vi "INIT SetPortProperties.vi"(8 "error in (no error)":errorcluster, 11 "Device Item Ref in":T1 format="%.0x") -> (0 "error out":errorcluster, 3 "Device Item Ref out":T1 format="%.0x")   [LabVIEW 2018, in "CAN Gateway System Explorer.lvlib"]
uses:
  CAN Gateway System Explorer.lvlib
  <vilib>/NI Veristand/Custom Device API/Custom Device Item Ref.ctl
  Shared/Constants.vi
  <vilib>/NI Veristand/Custom Device API/Set Item Property (String).vi
  <vilib>/NI Veristand/Custom Device API/Custom Device API.lvlib
  Shared/CAN Gateway Shared.lvlib
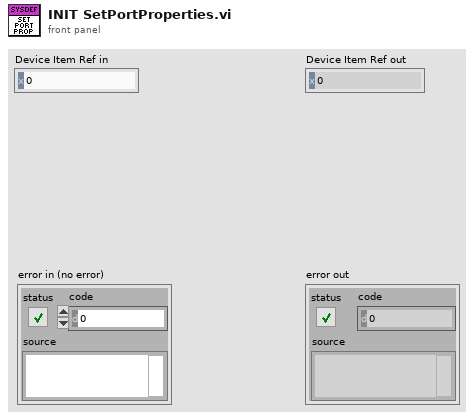
[diagram p1: front panel]
types:
  T1 = typedef "Custom Device API.lvlib/Custom Device Item Ref.ctl" = u64
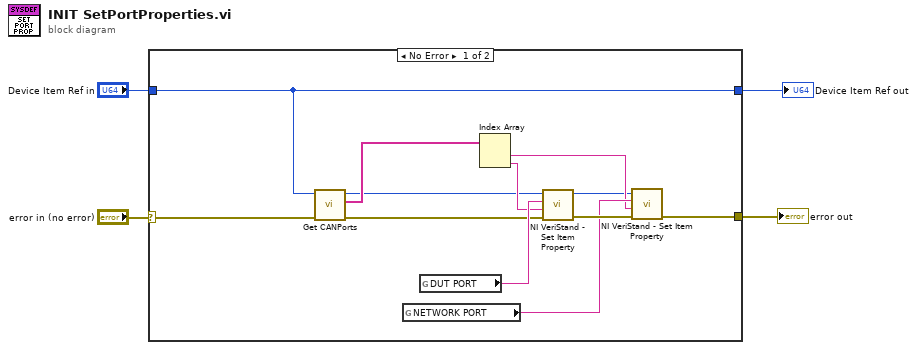
[diagram p0: block diagram]
diagram:
  n1 = case shown="No Error" "error in (no error)" {
    selector: "error in (no error)" -> [w16 w17]
    tunnel: "Device Item Ref in" -> [w8 w18]
    tunnel: [w9 w17] -> w2
    tunnel: [w8 w18] -> w1
    frame No Error {
      n2 = call "Get CANPorts.vi"("error in (no error)"=w16, "Device Item Ref in"=w8) -> ("error out"=w5:errorcluster, "CAN Ports"=w14:string[], "Device Item Ref out"=w6:T1)  [unwired: 7 in]
      n3 = global read "Constants.vi" "NETWORK PORT"() -> (w12:string)
      n4 = global read "Constants.vi" "DUT PORT"() -> (w15:string)
      n5 = Index Array(array=w14) -> (element #1=w10:string, element #2=w11:string)  [unwired: 2 in]
      n6 = call-poly <vilib>:"NI VeriStand - Set Item Property.vi"("error in (no error)"=w5, "Value"=w11, "Property Name"=w15, "Item Ref in"=w6) -> ("error out"=w13:errorcluster, "Item Ref out"=w7:T1)  [unwired: 5 in, 1 out]
      n7 = call-poly <vilib>:"NI VeriStand - Set Item Property.vi"("error in (no error)"=w13, "Value"=w10, "Property Name"=w12, "Item Ref in"=w7) -> ("error out"=w9:errorcluster)  [unwired: 5 in, 2 out]
    }
    frame Error {
    }
  }
  "error out" <- w2
  "Device Item Ref out" <- w1
